vi "Parse JSON.vi"(6 "error in (no error)":errorcluster, 8 "element":string, 9 "Data In":T1={"UI References"={"Exit Ref"=refnum, "Save Ref"=refnum, "Open Ref"=refnum, "Export Ref"=refnum, "Acquire Ref"=refnum, "Configure Ref"=refnum, "Graph Ref"=refnum, "Clear Ref"=refnum, "Analyze Ref"=refnum, "Status Ref"=refnum, "Snapshot Ref"=refnum}, "User Specified"={"Hardware Configuration"={"Signal Channel"="PXI1Slot7/ao0", "Response Channel"="PXI1Slot7/ai0", "Trigger Channel"="/PXI1Slot7/PFI0", "Number of Acquisitions"=1.0}, "Analysis Configuration"={"Statistics"=TRUE}, "Signal Type"=enum."From Excel", "New Data Behavior"=enum."Replace", "Signal Configuration"={"Chirp Amplitude"=0.0, "I/O Limit"=0.0, "Sample Rate"=0.0, "Chirp Duration (s)"=0.0, "Upper Frequency"=0.0, "Lower Frequency"=0.0, "Windowing"=enum."None"}, "Waveform File"="", "Save Location"=""}}) -> (0 "error out":errorcluster, 2 "States":T8=enum."Acquire", 3 "Data Out":T1={"UI References"={"Exit Ref"=refnum, "Save Ref"=refnum, "Open Ref"=refnum, "Export Ref"=refnum, "Acquire Ref"=refnum, "Configure Ref"=refnum, "Graph Ref"=refnum, "Clear Ref"=refnum, "Analyze Ref"=refnum, "Status Ref"=refnum, "Snapshot Ref"=refnum}, "User Specified"={"Hardware Configuration"={"Signal Channel"="PXI1Slot7/ao0", "Response Channel"="PXI1Slot7/ai0", "Trigger Channel"="/PXI1Slot7/PFI0", "Number of Acquisitions"=1.0}, "Analysis Configuration"={"Statistics"=TRUE}, "Signal Type"=enum."From Excel", "New Data Behavior"=enum."Replace", "Signal Configuration"={"Chirp Amplitude"=0.0, "I/O Limit"=0.0, "Sample Rate"=0.0, "Chirp Duration (s)"=0.0, "Upper Frequency"=0.0, "Lower Frequency"=0.0, "Windowing"=enum."None"}, "Waveform File"="", "Save Location"=""}}, 5 "channel":T7)   [LabVIEW 2017]
uses:
  controls/State.ctl
  <extravilib>/ChannelInstances/Event Messenger-c(a[.](str),t'Data.ctl')/))Channel.ctl
  controls/Data.ctl
  controls/UI References.ctl
  controls/HW Configuration.ctl
  controls/Analysis Configuration.ctl
  controls/New Data Behavior.ctl
  controls/Signal Configuration.ctl
  <extravilib>/ChannelInstances/Event Messenger-c(a[.](str),t'Data.ctl')/))Channel.vi
  <extravilib>/ChannelInstances/Event Messenger-c(a[.](str),t'Data.ctl').lvlib
panel:
  out "value":string
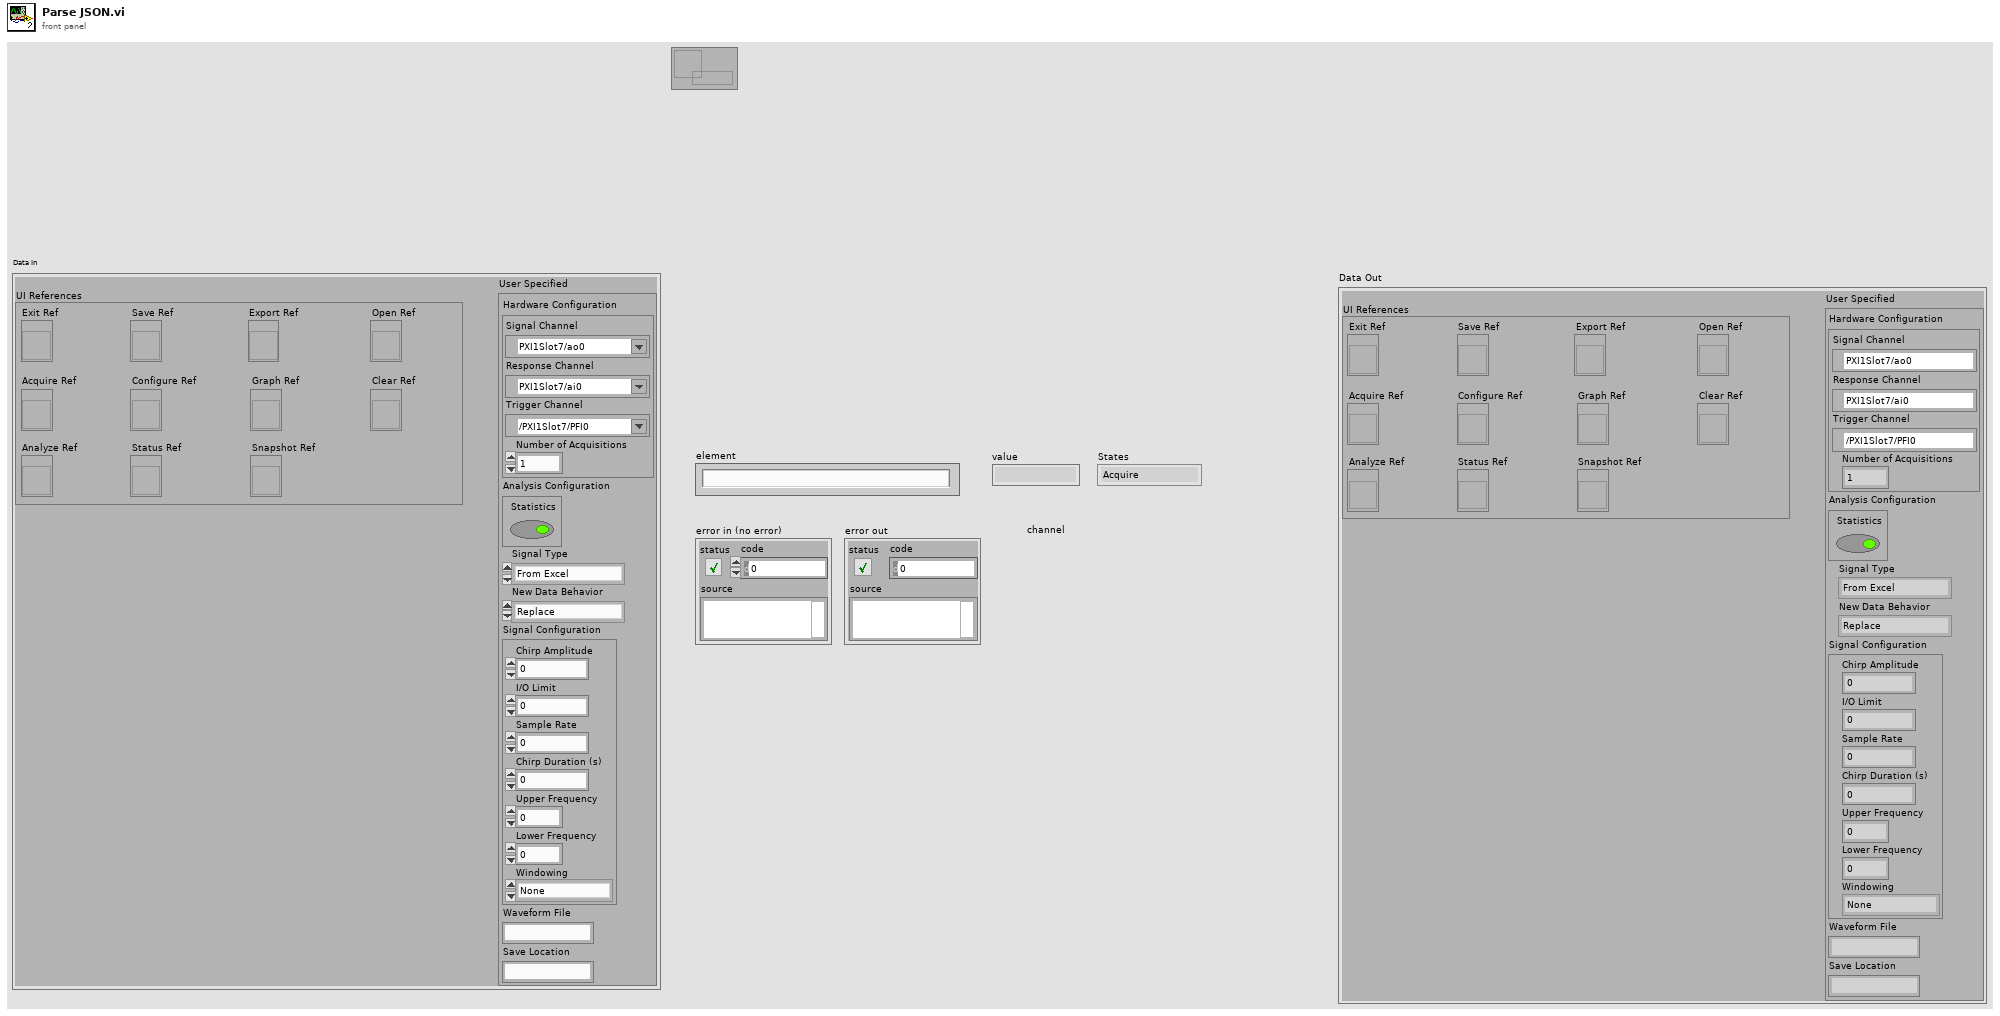
[diagram p1: front panel]
types:
  T1 = typedef "Data.ctl" = cluster{"UI References":T2, "User Specified":cluster{"Hardware Configuration":T3, "Analysis Configuration":T4, "Signal Type":enum16{"From Excel", "Single Chirp"}, "New Data Behavior":T5, "Signal Configuration":T6, "Waveform File":string, "Save Location":string}}
  T2 = typedef "UI References.ctl" = cluster{"Exit Ref":refnum<vi>, "Save Ref":refnum<vi>, "Open Ref":refnum<vi>, "Export Ref":refnum<vi>, "Acquire Ref":refnum<vi>, "Configure Ref":refnum<vi>, "Graph Ref":refnum<vi>, "Clear Ref":refnum<vi>, "Analyze Ref":refnum<vi>, "Status Ref":refnum<vi>, "Snapshot Ref":refnum<vi>}
  T3 = typedef "HW Configuration.ctl" = cluster{"Signal Channel":tag, "Response Channel":tag, "Trigger Channel":tag, "Number of Acquisitions":dbl}
  T4 = typedef "Analysis Configuration.ctl" = cluster{"Statistics":bool}
  T5 = typedef "New Data Behavior.ctl" = enum16{"Replace", "Overlay", "Append"}
  T6 = typedef "Signal Configuration.ctl" = cluster{"Chirp Amplitude":dbl, "I/O Limit":dbl, "Sample Rate":dbl, "Chirp Duration (s)":dbl, "Upper Frequency":dbl, "Lower Frequency":dbl, "Windowing":enum16{"None", "Exponential", "Flat top", "Hamming", "Hanning", "Kaiser-Bessel", "Rectangular"}}
  T7 = typedef "Event Messenger-c(a[.](str),t'Data.ctl').lvlib/))Channel.ctl" = refnum<queue>
  T8 = typedef "State.ctl" = enum16{"Initialize", "Wait for Event", "Update UI", "Configure", "Acquire", "Load Data", "Save Data", "Clear Data", "Export Data", "Analyze", "Copy Graph", "Exit"}
  T9 = enum16{"None", "Exponential", "Flat top", "Hamming", "Hanning", "Kaiser-Bessel", "Rectangular"}
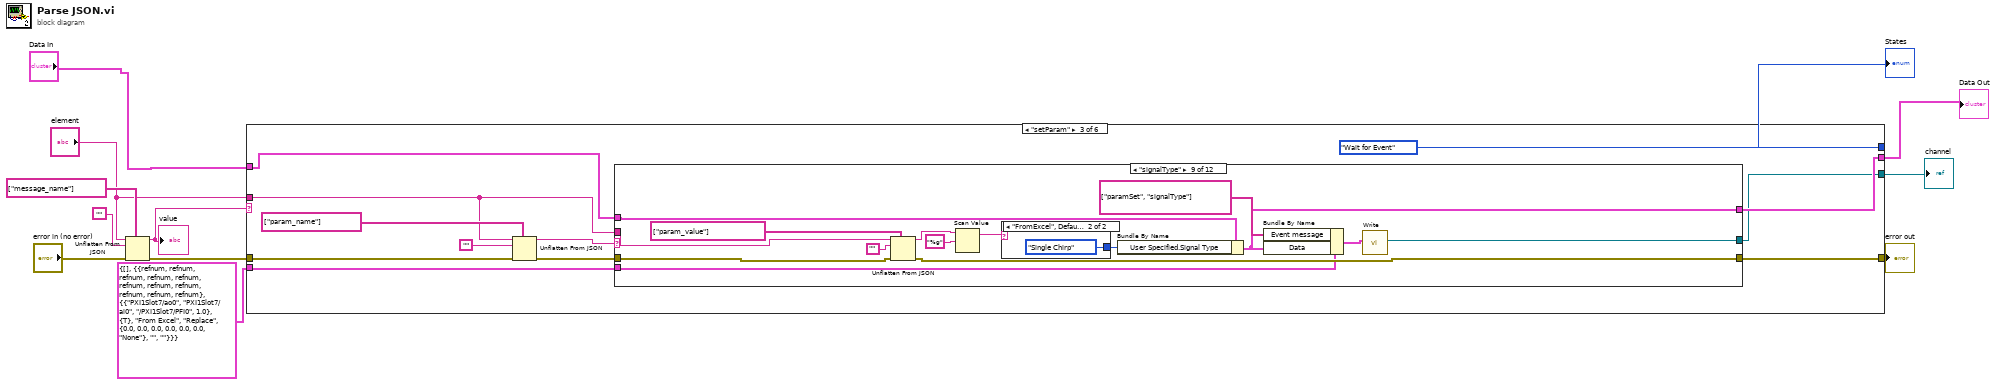
[diagram p0: block diagram]
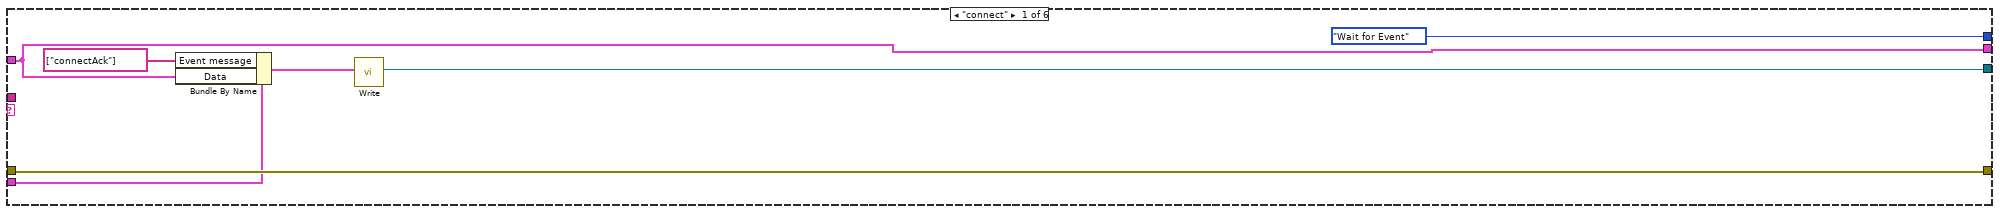
[diagram p2: hidden frame]
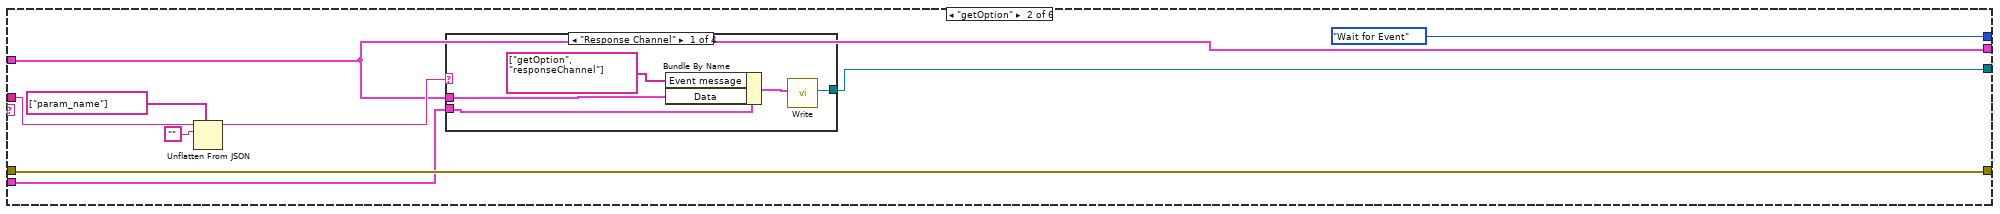
[diagram p3: hidden frame]
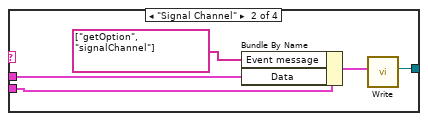
[diagram p4: hidden frame]
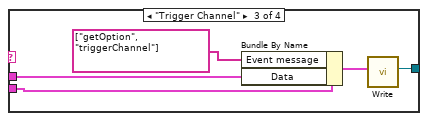
[diagram p5: hidden frame]
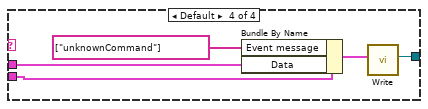
[diagram p6: hidden frame]
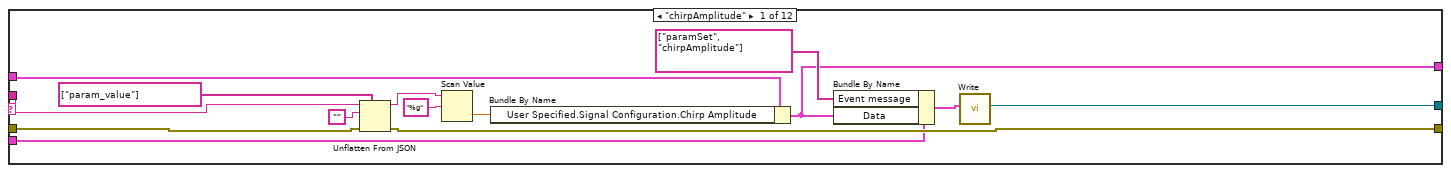
[diagram p7: hidden frame]
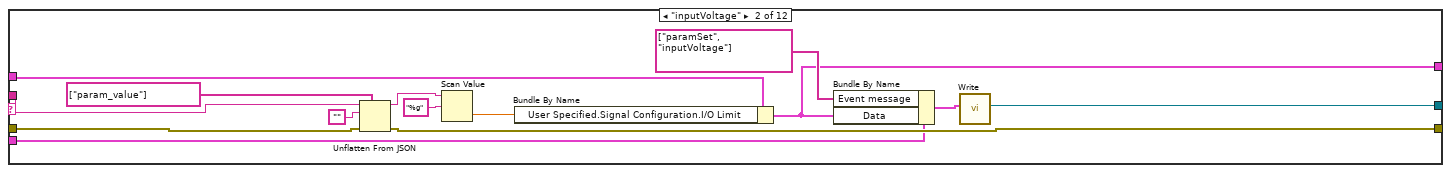
[diagram p8: hidden frame]
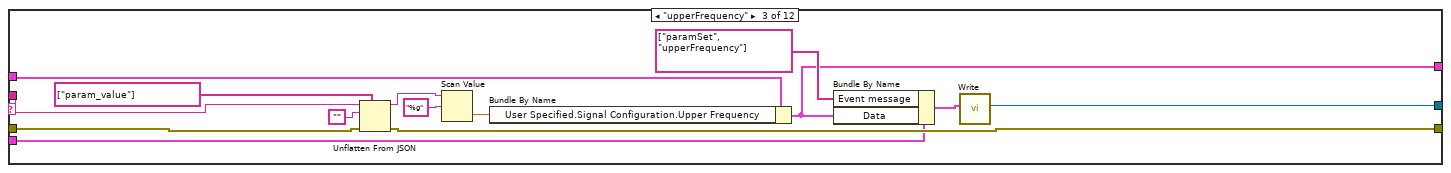
[diagram p9: hidden frame]
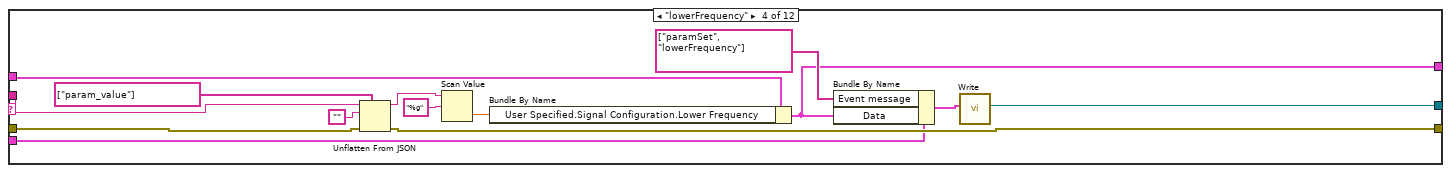
[diagram p10: hidden frame]
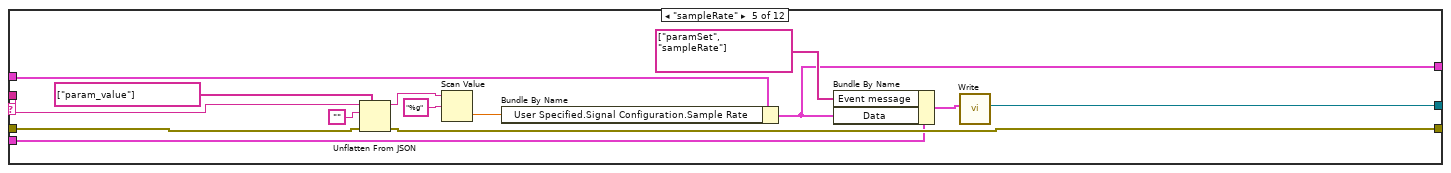
[diagram p11: hidden frame]
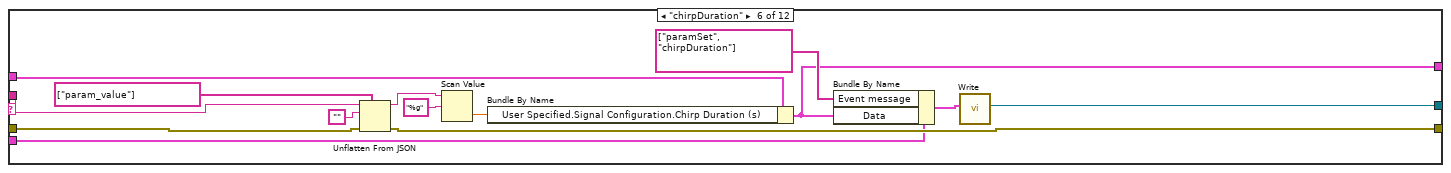
[diagram p12: hidden frame]
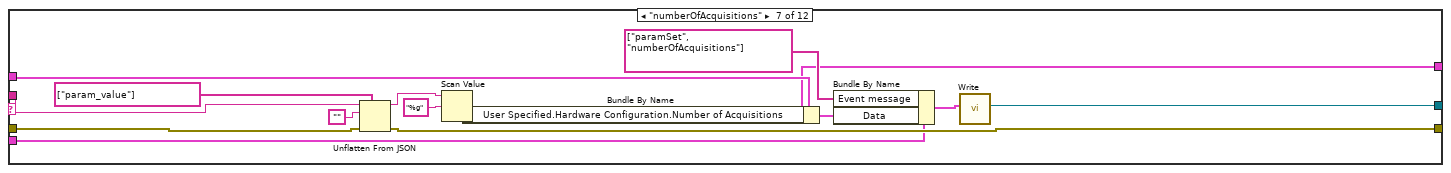
[diagram p13: hidden frame]
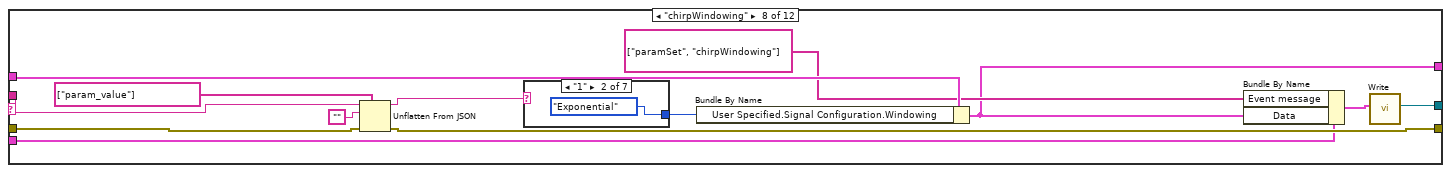
[diagram p14: hidden frame]
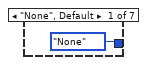
[diagram p15: hidden frame]
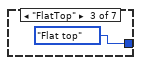
[diagram p16: hidden frame]
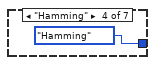
[diagram p17: hidden frame]
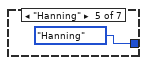
[diagram p18: hidden frame]
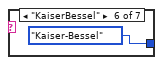
[diagram p19: hidden frame]
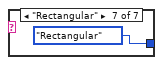
[diagram p20: hidden frame]
diagram:
  n1 = Unflatten From JSON(path=string[] ["message_name"], JSON string="element", type and defaults="", error in (no error)="error in (no error)") -> (value=w9:string, error out=w7:errorcluster)  [unwired: 3 in]
  "value" <- w9
  n2 = case shown="\"setParam\"" w9 {
    tunnel: "element" -> [_ w28 w56 _ _ _]
    tunnel: w7 -> [w19 w26 w57 w236 w243 w249]
    tunnel: [w13 w20 w53 w230 w237 w244] -> w1
    tunnel: [w19 w26 w54 w236 w243 w249] -> w6
    tunnel: [State."Wait for Event" ("States") State."Wait for Event" ("States") State."Wait for Event" ("States") State."Acquire" ("States") State."Exit" ("States") State."Wait for Event" ("States")] -> w5
    tunnel: cluster{"Event message":string[], "Data":T1} {"Event message"=[], "Data"={"UI References"={"Exit Ref"=refnum, "Save Ref"=refnum, "Open Ref"=refnum, "Export Ref"=refnum, "Acquire Ref"=refnum, "Configure Ref"=refnum, "Graph Ref"=refnum, "Clear Ref"=refnum, "Analyze Ref"=refnum, "Status Ref"=refnum, "Snapshot Ref"=refnum}, "User Specified"={"Hardware Configuration"={"Signal Channel"="PXI1Slot7/ao0", "Response Channel"="PXI1Slot7/ai0", "Trigger Channel"="/PXI1Slot7/PFI0", "Number of Acquisitions"=1.0}, "Analysis Configuration"={"Statistics"=TRUE}, "Signal Type"=enum."From Excel", "New Data Behavior"=enum."Replace", "Signal Configuration"={"Chirp Amplitude"=0.0, "I/O Limit"=0.0, "Sample Rate"=0.0, "Chirp Duration (s)"=0.0, "Upper Frequency"=0.0, "Lower Frequency"=0.0, "Windowing"=enum."None"}, "Waveform File"="", "Save Location"=""}}} -> [w15 w22 w51 w234 w241 w247]
    tunnel: [w14 w21 w50 w231 w238 w245] -> w3
    tunnel: "Data In" -> [w13 w20 w49 w230 w237 w244]
    frame "connect" {
      n3 = Bundle By Name(cluster=w15, "Event message"=string[] ["connectAck"], "Data"=w13) -> (w17:cluster{"Event message":string[], "Data":T1})
      n4 = call <extravilib>:"Write.vi"("element"=w17) -> ("channel"=w14:T7)  [unwired: 9 in, 1 out]
    }
    frame "getOption" {
      n5 = Unflatten From JSON(path=string[] ["param_name"], JSON string=w28, type and defaults="") -> (value=w25:string)  [unwired: 4 in, 1 out]
      n6 = case shown="\"Response Channel\"" w25 {
        tunnel: w22 -> [w31 w36 w41 w46]
        tunnel: w20 -> [w32 w37 w42 w45]
        tunnel: [w29 w38 w39 w44] -> w21
        frame "Response Channel" {
          n7 = Bundle By Name(cluster=w31, "Event message"=string[] ["getOption", "responseChannel"], "Data"=w32) -> (w30:cluster{"Event message":string[], "Data":T1})
          n8 = call <extravilib>:"Write.vi"("element"=w30) -> ("channel"=w29:T7)  [unwired: 9 in, 1 out]
        }
        frame "Signal Channel" {
          n9 = Bundle By Name(cluster=w36, "Event message"=string[] ["getOption", "signalChannel"], "Data"=w37) -> (w34:cluster{"Event message":string[], "Data":T1})
          n10 = call <extravilib>:"Write.vi"("element"=w34) -> ("channel"=w38:T7)  [unwired: 9 in, 1 out]
        }
        frame "Trigger Channel" {
          n11 = Bundle By Name(cluster=w41, "Event message"=string[] ["getOption", "triggerChannel"], "Data"=w42) -> (w40:cluster{"Event message":string[], "Data":T1})
          n12 = call <extravilib>:"Write.vi"("element"=w40) -> ("channel"=w39:T7)  [unwired: 9 in, 1 out]
        }
        frame Default {
          n13 = Bundle By Name(cluster=w46, "Event message"=string[] ["unknownCommand"], "Data"=w45) -> (w48:cluster{"Event message":string[], "Data":T1})
          n14 = call <extravilib>:"Write.vi"("element"=w48) -> ("channel"=w44:T7)  [unwired: 9 in, 1 out]
        }
      }
    }
    frame "setParam" {
      n15 = Unflatten From JSON(path=string[] ["param_name"], JSON string=w56, type and defaults="", error in (no error)=w57) -> (value=w58:string, error out=w55:errorcluster)  [unwired: 3 in]
      n16 = case shown="\"signalType\"" w58 {
        tunnel: w56 -> [w73 w87 w101 w115 w129 w143 w157 w170 w192 w208 w222 _]
        tunnel: w49 -> [w72 w86 w100 w114 w128 w142 w156 w169 w191 w207 w221 w225]
        tunnel: [w63 w78 w91 w105 w120 w134 w148 w163 w184 w200 w214 w225] -> w53
        tunnel: w55 -> [w71 w85 w99 w113 w127 w141 w155 w168 w190 w206 w220 w229]
        tunnel: [w70 w84 w98 w112 w126 w140 w154 w167 w189 w205 w219 w229] -> w54
        tunnel: w51 -> [w66 w79 w94 w107 w122 w133 w147 w162 w183 w199 w213 w228]
        tunnel: [w62 w76 w90 w104 w118 w136 w150 w165 w186 w202 w216 w224] -> w50
        frame "chirpAmplitude" {
          n17 = Unflatten From JSON(path=string[] ["param_value"], JSON string=w73, type and defaults="", error in (no error)=w71) -> (value=w68:string, error out=w70:errorcluster)  [unwired: 3 in]
          n18 = Scan Value(string=w68, format string="%g") -> (value=w67:dbl)  [unwired: 1 in, 1 out]
          n19 = Bundle By Name(cluster=w72, "User Specified.Signal Configuration.Chirp Amplitude"=w67) -> (w63:T1)
          n20 = Bundle By Name(cluster=w66, "Event message"=string[] ["paramSet", "chirpAmplitude"], "Data"=w63) -> (w65:cluster{"Event message":string[], "Data":T1})
          n21 = call <extravilib>:"Write.vi"("element"=w65) -> ("channel"=w62:T7)  [unwired: 9 in, 1 out]
        }
        frame "inputVoltage" {
          n22 = Unflatten From JSON(path=string[] ["param_value"], JSON string=w87, type and defaults="", error in (no error)=w85) -> (value=w83:string, error out=w84:errorcluster)  [unwired: 3 in]
          n23 = Scan Value(string=w83, format string="%g") -> (value=w82:dbl)  [unwired: 1 in, 1 out]
          n24 = Bundle By Name(cluster=w86, "User Specified.Signal Configuration.I/O Limit"=w82) -> (w78:T1)
          n25 = Bundle By Name(cluster=w79, "Event message"=string[] ["paramSet", "inputVoltage"], "Data"=w78) -> (w77:cluster{"Event message":string[], "Data":T1})
          n26 = call <extravilib>:"Write.vi"("element"=w77) -> ("channel"=w76:T7)  [unwired: 9 in, 1 out]
        }
        frame "upperFrequency" {
          n27 = Unflatten From JSON(path=string[] ["param_value"], JSON string=w101, type and defaults="", error in (no error)=w99) -> (value=w96:string, error out=w98:errorcluster)  [unwired: 3 in]
          n28 = Scan Value(string=w96, format string="%g") -> (value=w95:dbl)  [unwired: 1 in, 1 out]
          n29 = Bundle By Name(cluster=w100, "User Specified.Signal Configuration.Upper Frequency"=w95) -> (w91:T1)
          n30 = Bundle By Name(cluster=w94, "Event message"=string[] ["paramSet", "upperFrequency"], "Data"=w91) -> (w93:cluster{"Event message":string[], "Data":T1})
          n31 = call <extravilib>:"Write.vi"("element"=w93) -> ("channel"=w90:T7)  [unwired: 9 in, 1 out]
        }
        frame "lowerFrequency" {
          n32 = Unflatten From JSON(path=string[] ["param_value"], JSON string=w115, type and defaults="", error in (no error)=w113) -> (value=w109:string, error out=w112:errorcluster)  [unwired: 3 in]
          n33 = Scan Value(string=w109, format string="%g") -> (value=w110:dbl)  [unwired: 1 in, 1 out]
          n34 = Bundle By Name(cluster=w114, "User Specified.Signal Configuration.Lower Frequency"=w110) -> (w105:T1)
          n35 = Bundle By Name(cluster=w107, "Event message"=string[] ["paramSet", "lowerFrequency"], "Data"=w105) -> (w108:cluster{"Event message":string[], "Data":T1})
          n36 = call <extravilib>:"Write.vi"("element"=w108) -> ("channel"=w104:T7)  [unwired: 9 in, 1 out]
        }
        frame "sampleRate" {
          n37 = Unflatten From JSON(path=string[] ["param_value"], JSON string=w129, type and defaults="", error in (no error)=w127) -> (value=w124:string, error out=w126:errorcluster)  [unwired: 3 in]
          n38 = Scan Value(string=w124, format string="%g") -> (value=w123:dbl)  [unwired: 1 in, 1 out]
          n39 = Bundle By Name(cluster=w128, "User Specified.Signal Configuration.Sample Rate"=w123) -> (w120:T1)
          n40 = Bundle By Name(cluster=w122, "Event message"=string[] ["paramSet", "sampleRate"], "Data"=w120) -> (w119:cluster{"Event message":string[], "Data":T1})
          n41 = call <extravilib>:"Write.vi"("element"=w119) -> ("channel"=w118:T7)  [unwired: 9 in, 1 out]
        }
        frame "chirpDuration" {
          n42 = Unflatten From JSON(path=string[] ["param_value"], JSON string=w143, type and defaults="", error in (no error)=w141) -> (value=w138:string, error out=w140:errorcluster)  [unwired: 3 in]
          n43 = Scan Value(string=w138, format string="%g") -> (value=w137:dbl)  [unwired: 1 in, 1 out]
          n44 = Bundle By Name(cluster=w142, "User Specified.Signal Configuration.Chirp Duration (s)"=w137) -> (w134:T1)
          n45 = Bundle By Name(cluster=w133, "Event message"=string[] ["paramSet", "chirpDuration"], "Data"=w134) -> (w132:cluster{"Event message":string[], "Data":T1})
          n46 = call <extravilib>:"Write.vi"("element"=w132) -> ("channel"=w136:T7)  [unwired: 9 in, 1 out]
        }
        frame "numberOfAcquisitions" {
          n47 = Unflatten From JSON(path=string[] ["param_value"], JSON string=w157, type and defaults="", error in (no error)=w155) -> (value=w152:string, error out=w154:errorcluster)  [unwired: 3 in]
          n48 = Scan Value(string=w152, format string="%g") -> (value=w151:dbl)  [unwired: 1 in, 1 out]
          n49 = Bundle By Name(cluster=w156, "User Specified.Hardware Configuration.Number of Acquisitions"=w151) -> (w148:T1)
          n50 = Bundle By Name(cluster=w147, "Event message"=string[] ["paramSet", "numberOfAcquisitions"], "Data"=w148) -> (w146:cluster{"Event message":string[], "Data":T1})
          n51 = call <extravilib>:"Write.vi"("element"=w146) -> ("channel"=w150:T7)  [unwired: 9 in, 1 out]
        }
        frame "chirpWindowing" {
          n52 = Unflatten From JSON(path=string[] ["param_value"], JSON string=w170, type and defaults="", error in (no error)=w168) -> (value=w159:string, error out=w167:errorcluster)  [unwired: 3 in]
          n53 = case shown="\"1\"" w159 {
            tunnel: [T9."None" ("User Specified.Signal Configuration.Windowing") T9."Exponential" ("User Specified.Signal Configuration.Windowing") T9."Flat top" ("User Specified.Signal Configuration.Windowing") T9."Hamming" ("User Specified.Signal Configuration.Windowing") T9."Hanning" ("User Specified.Signal Configuration.Windowing") T9."Kaiser-Bessel" ("User Specified.Signal Configuration.Windowing") T9."Rectangular" ("User Specified.Signal Configuration.Windowing")] -> w160
            frame "None", Default {
            }
            frame "1" {
            }
            frame "FlatTop" {
            }
            frame "Hamming" {
            }
            frame "Hanning" {
            }
            frame "KaiserBessel" {
            }
            frame "Rectangular" {
            }
          }
          n54 = Bundle By Name(cluster=w169, "User Specified.Signal Configuration.Windowing"=w160) -> (w163:T1)
          n55 = Bundle By Name(cluster=w162, "Event message"=string[] ["paramSet", "chirpWindowing"], "Data"=w163) -> (w161:cluster{"Event message":string[], "Data":T1})
          n56 = call <extravilib>:"Write.vi"("element"=w161) -> ("channel"=w165:T7)  [unwired: 9 in, 1 out]
        }
        frame "signalType" {
          n57 = Unflatten From JSON(path=string[] ["param_value"], JSON string=w192, type and defaults="", error in (no error)=w190) -> (value=w187:string, error out=w189:errorcluster)  [unwired: 3 in]
          n58 = Scan Value(string=w187, format string="%g") -> (output string=w180:string)  [unwired: 1 in, 1 out]
          n59 = case shown="\"FromExcel\", Default" w180 {
            tunnel: [enum16{"Single Chirp", "From Excel"}."Single Chirp" ("User Specified.Signal Type") enum16{"From Excel", "Single Chirp"}."Single Chirp" ("User Specified.Signal Type")] -> w179
            frame "SingleChirp" {
            }
            frame "FromExcel", Default {
            }
          }
          n60 = Bundle By Name(cluster=w191, "User Specified.Signal Type"=w179) -> (w184:T1)
          n61 = Bundle By Name(cluster=w183, "Event message"=string[] ["paramSet", "signalType"], "Data"=w184) -> (w182:cluster{"Event message":string[], "Data":T1})
          n62 = call <extravilib>:"Write.vi"("element"=w182) -> ("channel"=w186:T7)  [unwired: 9 in, 1 out]
        }
        frame "waveformSpecificationFile" {
          n63 = Unflatten From JSON(path=string[] ["param_value"], JSON string=w208, type and defaults="", error in (no error)=w206) -> (value=w203:string, error out=w205:errorcluster)  [unwired: 3 in]
          n64 = Scan Value(string=w203, format string="%g") -> (output string=w196:string)  [unwired: 1 in, 1 out]
          n65 = Bundle By Name(cluster=w207, "User Specified.Waveform File"=w196) -> (w200:T1)
          n66 = Bundle By Name(cluster=w199, "Event message"=string[] ["paramSet", "waveformSpecificationFile"], "Data"=w200) -> (w198:cluster{"Event message":string[], "Data":T1})
          n67 = call <extravilib>:"Write.vi"("element"=w198) -> ("channel"=w202:T7)  [unwired: 9 in, 1 out]
        }
        frame "saveLocation" {
          n68 = Unflatten From JSON(path=string[] ["param_value"], JSON string=w222, type and defaults="", error in (no error)=w220) -> (value=w217:string, error out=w219:errorcluster)  [unwired: 3 in]
          n69 = Scan Value(string=w217, format string="%g") -> (output string=w210:string)  [unwired: 1 in, 1 out]
          n70 = Bundle By Name(cluster=w221, "User Specified.Save Location"=w210) -> (w214:T1)
          n71 = Bundle By Name(cluster=w213, "Event message"=string[] ["paramSet", "saveLocation"], "Data"=w214) -> (w212:cluster{"Event message":string[], "Data":T1})
          n72 = call <extravilib>:"Write.vi"("element"=w212) -> ("channel"=w216:T7)  [unwired: 9 in, 1 out]
        }
        frame Default {
          n73 = Bundle By Name(cluster=w228, "Event message"=string[] ["unknownCommand"], "Data"=w225) -> (w227:cluster{"Event message":string[], "Data":T1})
          n74 = call <extravilib>:"Write.vi"("element"=w227) -> ("channel"=w224:T7)  [unwired: 9 in, 1 out]
        }
      }
    }
    frame "startExperiment" {
      n75 = Bundle By Name(cluster=w234, "Event message"=string[] ["experimentStarted"], "Data"=w230) -> (w232:cluster{"Event message":string[], "Data":T1})
      n76 = call <extravilib>:"Write.vi"("element"=w232) -> ("channel"=w231:T7)  [unwired: 9 in, 1 out]
    }
    frame "stopExperiment" {
      n77 = Bundle By Name(cluster=w241, "Event message"=string[] ["experimentStopped"], "Data"=w237) -> (w240:cluster{"Event message":string[], "Data":T1})
      n78 = call <extravilib>:"Write.vi"("element"=w240) -> ("channel"=w238:T7)  [unwired: 9 in, 1 out]
    }
    frame Default {
      n79 = Bundle By Name(cluster=w247, "Event message"=string[] ["unknownCommand"], "Data"=w244) -> (w246:cluster{"Event message":string[], "Data":T1})
      n80 = call <extravilib>:"Write.vi"("element"=w246) -> ("channel"=w245:T7)  [unwired: 9 in, 1 out]
    }
  }
  "States" <- w5
  "error out" <- w6
  "channel" <- w3
  "Data Out" <- w1
